vi "Run Top Level.vi"(6 "Variant in":variant, 7 "Shift Pressed?":bool, 8 "error in":errorcluster, 10 "QD Combo Box Ref":refnum<vi>, 11 "QD Launch VI Ref":refnum<vi>) -> (0 "error out":errorcluster, 4 "Variant out":variant)   [LabVIEW 2020]
doc: "Run the top level VI in the project.\n\nDefault Shortcut - [E]"
panel:
  in  "Undo Name":string="Quick Drop Keyboard Shortcut"
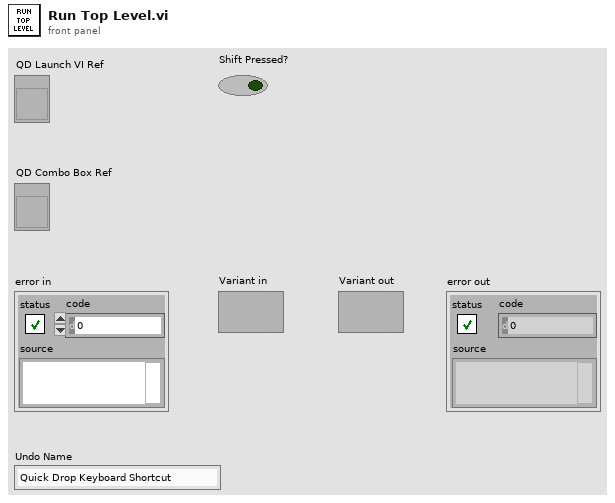
[diagram p1: front panel]
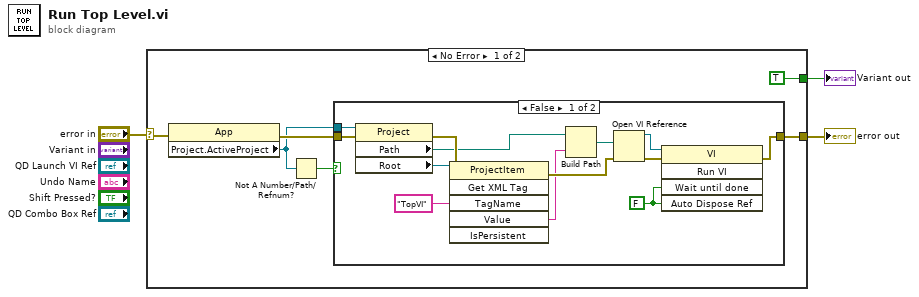
[diagram p0: block diagram]
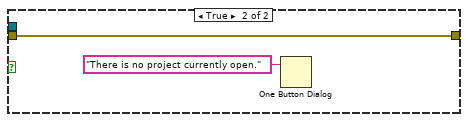
[diagram p2: hidden frame]
diagram:
  n1 = case shown="No Error" "error in" {
    selector: "error in" -> [w7 w25]
    tunnel: [w8 w25] -> w2
    tunnel: [TRUE _] -> w1
    frame No Error {
      n2 = property class="App"(error in=w7) -> (error out=w9:errorcluster, "Project.ActiveProject"=w5:refnum<vi>)  [unwired: 1 in, 1 out]
      n3 = Not A Number/Path/Refnum?(number/path/refnum=w5) -> (NaN/Path/Refnum?=w4:bool)
      n4 = case shown="False" w4 {
        tunnel: w9 -> [w22 w24]
        tunnel: [w18 w24] -> w8
        tunnel: w5 -> [w17 _]
        frame False {
          w13 = FALSE ("Auto Dispose Reference")
          n5 = property class="Project"(reference=w17, error in=w22) -> (error out=w21:errorcluster, "Path"=w12:path, "Root"=w15:refnum<vi>)  [unwired: 1 out]
          n6 = invoke class="ProjectItem" method="Get XML Tag"(reference=w15, error in=w21, "TagName"="TopVI" ("Tag Name")) -> (error out=w20:errorcluster, "Value"=w11:string)  [unwired: 3 in, 4 out]
          n7 = Build Path(base path=w12, name or relative path=w11) -> (appended path=w10:path)
          n8 = Open VI Reference(vi path=w10, error in (no error)=w20) -> (vi reference=w14:refnum<vi>, error out=w19:errorcluster)  [unwired: 4 in]
          n9 = invoke class="VI" method="Run VI"(reference=w14, error in=w19, "Wait until done"=w13, "Auto Dispose Ref"=w13) -> (error out=w18:errorcluster)  [unwired: 1 in, 4 out]
        }
        frame True {
          n10 = One Button Dialog(message="There is no project currently open.") -> ()  [unwired: 1 in, 1 out]
        }
      }
    }
    frame Error {
    }
  }
  "error out" <- w2
  "Variant out" <- w1
